vi "MSEncoder Case-20-UpdAuxArbPulses.vi"(8 "error in (no error)":errorcluster, 9 "ParamValIn":variant, 11 "MSEncoder in":refnum<class "MSEncoder.lvclass">) -> (0 "error out":errorcluster, 3 "MSEncoder out":refnum<class "MSEncoder.lvclass">)   [LabVIEW 2018, in "MSEncoder.lvclass"]
uses:
  MSEncoder.lvclass
  Ctl/MSEditorParam updAuxArbPulses.ctl
  MSEncoder.lvclass/MSEncoder.ctl
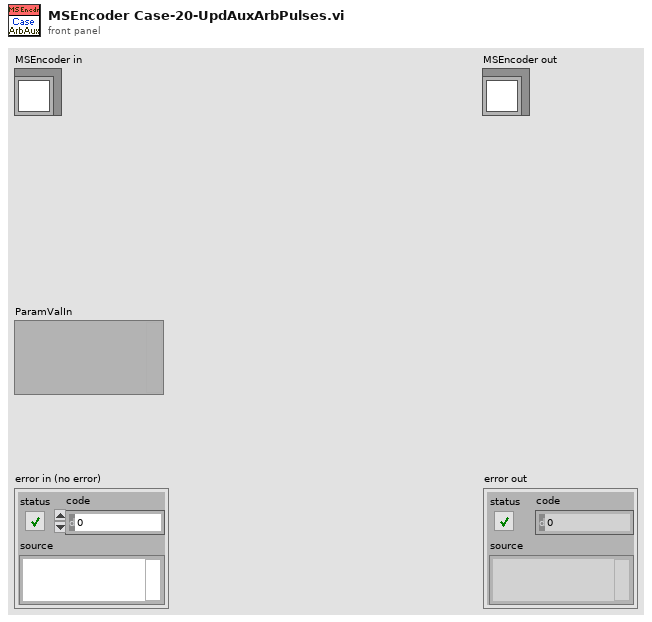
[diagram p1: front panel]
types:
  T1 = typedef "MSEditorParam updAuxArbPulses.ctl" = cluster{"cycleIni":ext[], "cycleEnd":ext[], "pulseInt":ext[]}
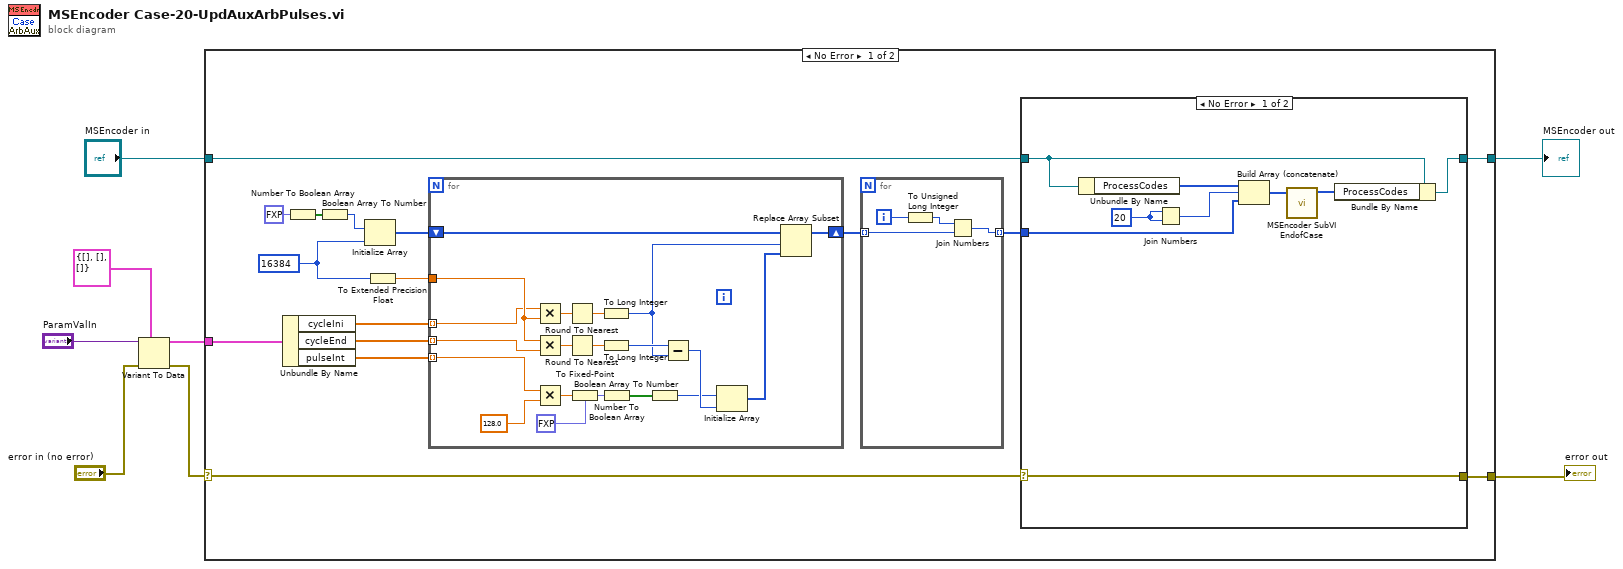
[diagram p0: block diagram]
diagram:
  n1 = Variant To Data(error in="error in (no error)", type=T1 {"cycleIni"=[], "cycleEnd"=[], "pulseInt"=[]}, Variant="ParamValIn") -> (data=w2:T1, error out=w3:errorcluster)
  n2 = case shown="No Error" w3 {
    selector: w3 -> [w16 w61]
    tunnel: "MSEncoder in" -> [w22 w60]
    tunnel: [w23 w61] -> w8
    tunnel: [w24 w60] -> w6
    tunnel: w2 -> [w13 _]
    frame No Error {
      w9 = 16384 ("dimension size")
      n3 = Unbundle By Name(w13) -> ("cycleIni"=w12:ext[], "cycleEnd"=w11:ext[], "pulseInt"=w10:ext[])
      n4 = Number To Boolean Array(number=fxp<+/-,9,9> 0.0) -> (Boolean array=w17:bool[])
      n5 = Boolean Array To Number(Boolean array=w17) -> (number=w18:u32)
      n6 = Initialize Array(w18, w9) -> (w21:u32[])
      n7 = To Extended Precision Float(1:w9) -> (0:w20:ext)
      n8 = for {
        tunnel: w20 -> [w48]
        shift-right: [w45] -> w15
        shift-left: w21 -> [w46]
        tunnel: w12 -> [w31] mode=indexing
        tunnel: w11 -> [w30] mode=indexing
        tunnel: w10 -> [w29] mode=indexing
        n9 = Multiply(x=w31, y=w48) -> (x*y=w42:ext)
        n10 = Multiply(x=w48, y=w30) -> (x*y=w41:ext)
        n11 = Multiply(x=w29, y=128.0 ("PulseInt")) -> (x*y=w44:ext)
        n12 = Round To Nearest(number=w42) -> (nearest integer value=w40:ext)
        n13 = Round To Nearest(number=w41) -> (nearest integer value=w39:ext)
        n14 = To Fixed-Point(fixed-point type=fxp<+/-,9,9> 0.0 ("new element/subarray"), number=w44) -> (fixed-point=w33:fxp<+/-,9,9>)
        n15 = To Long Integer(number=w40) -> (32bit integer=w37:i32)
        n16 = To Long Integer(number=w39) -> (32bit integer=w38:i32)
        n17 = Number To Boolean Array(number=w33) -> (Boolean array=w34:bool[])
        n18 = Boolean Array To Number(Boolean array=w34) -> (number=w32:u32)
        n19 = Subtract(x=w38, y=w37) -> (x-y=w36:i32)
        n20 = Initialize Array(w32, w36) -> (w35:u32[])
        n21 = Replace Array Subset(array=w46, new element=w35, index=w37) -> (w45:u32[])
      }
      n22 = for {
        tunnel: w15 -> [w26] mode=indexing
        tunnel: [w25] -> w14 mode=indexing
        i -> [w28]
        n23 = To Unsigned Long Integer(number=w28) -> (unsigned 32bit integer=w27:u32)
        n24 = Join Numbers(hi=w27, lo=w26) -> ((hi.lo)=w25:u64)
      }
      n25 = case shown="No Error" w16 {
        selector: w16 -> [w50 w59]
        tunnel: [w57 w58] -> w24
        tunnel: w22 -> [w51 w58]
        tunnel: [w50 w59] -> w23
        tunnel: w14 -> [w49 _]
        frame No Error {
          w53 = u32 20
          n26 = Unbundle By Name(w51) -> ("ProcessCodes"=w52:u64[])
          n27 = Join Numbers(hi=w53, lo=w53) -> ((hi.lo)=w56:u64)
          n28 = Build Array (concatenate)(w52, w56, w49) -> (w55:u64[])
          n29 = call "MSEncoder SubVI EndofCase.vi"("Case codes"=w55) -> ("Case codes with end"=w54:u64[])  [unwired: 9 in, 1 out]
          n30 = Bundle By Name(cluster=w51, "ProcessCodes"=w54) -> (w57:refnum<class "MSEncoder.lvclass">)
        }
        frame Error {
        }
      }
    }
    frame Error {
    }
  }
  "error out" <- w8
  "MSEncoder out" <- w6
